vi "Configuration--FGV.vi"(7 "Functional Global Action":T4, 9 "Module Number":i32, 10 "Module Configuration In":T2, 11 "Carrier Configuration In":T1) -> (2 "Module Configuration Out":T2, 3 "Carrier Configuration Out":T1)   [LabVIEW 2017, in "Communications Library.lvlib"]
doc: "Functional gloabl variable, which stores the current configuration of the DTACQ device. \n\nNote: Writting the carrier configuration will also replace the module configurations."
uses:
  Communications Library.lvlib
  Typedefs/Functional Global Variable Action--Enum.ctl
  Typedefs/DTACQ Module Carrier Configuration--Cluster.ctl
  Typedefs/DTACQ Module Configuration--Cluster.ctl
  Typedefs/DTACQ Device Type--Enum.ctl
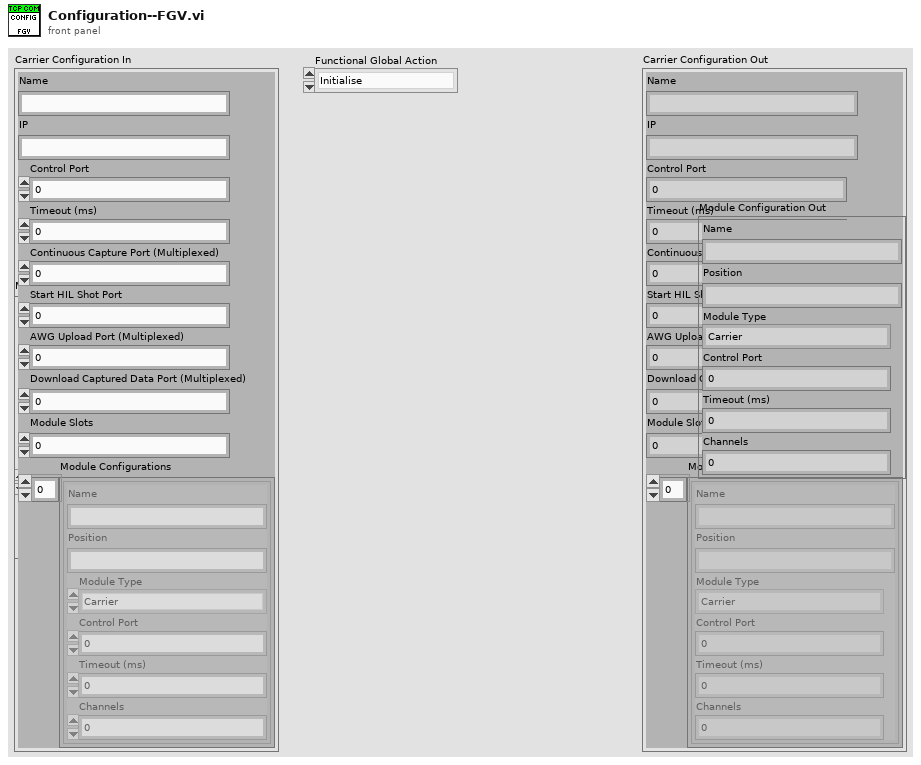
[diagram p1: front panel]
types:
  T1 = typedef "Communications Library.lvlib/DTACQ Module Carrier Configuration--Cluster.ctl" = cluster{"Name":string, "IP":string, "Control Port":i32, "Timeout (ms)":i32, "Continuous Capture Port (Multiplexed)":i32, "Start HIL Shot Port":i32, "AWG Upload Port (Multiplexed)":i32, "Download Captured Data Port (Multiplexed)":i32, "Module Slots":i32, "Module Configurations":T2[]}
  T2 = typedef "Communications Library.lvlib/DTACQ Module Configuration--Cluster.ctl" = cluster{"Name":string, "Position":string, "Module Type":T3, "Control Port":i32, "Timeout (ms)":i32, "Channels":i32}
  T3 = typedef "Communications Library.lvlib/DTACQ Device Type--Enum.ctl" = enum16{"Carrier", "Analog In Module", "Analog Out Module", "Generic Module"}
  T4 = typedef "Communications Library.lvlib/Functional Global Variable Action--Enum.ctl" = enum16{"Initialise", "Write Module Config", "Write Carrier Config", "Read"}
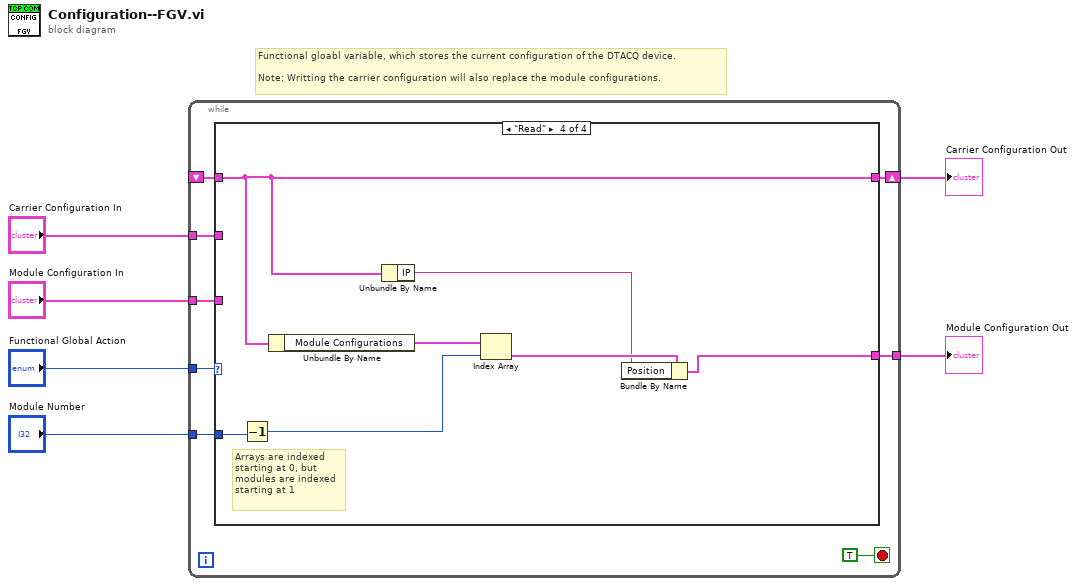
[diagram p0: block diagram]
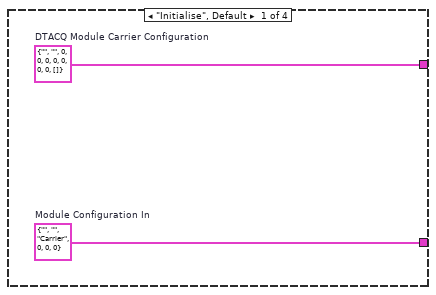
[diagram p2: hidden frame]
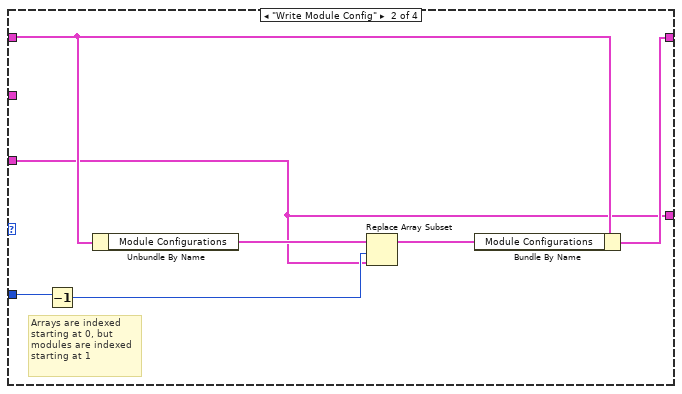
[diagram p3: hidden frame]
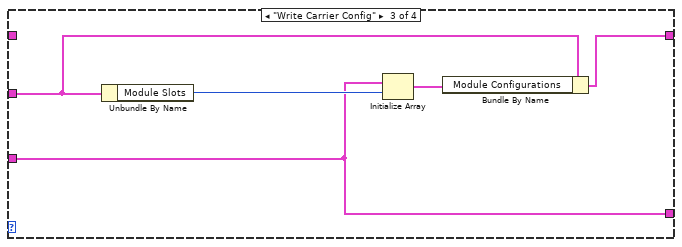
[diagram p4: hidden frame]
diagram:
  # "Functional gloabl variable, which stores the current configuration of the DTACQ device.  \n\nNote: Writting the carrier configuration will also replace the module configurations."
  n1 = while {
    tunnel: "Functional Global Action" -> [w14]
    shift-right: [w13] -> w4
    shift-left: _ -> [w12]
    tunnel: "Module Number" -> [w11]
    tunnel: [w10] -> w3
    tunnel: "Module Configuration In" -> [w9]
    tunnel: "Carrier Configuration In" -> [w8]
    stop <- TRUE stop-if-true
    n2 = case shown="\"Read\"" w14 {
      tunnel: [w16 w22 w25 w32] -> w13
      tunnel: w12 -> [_ w23 _ w32]
      tunnel: w11 -> [_ w20 _ w34]
      tunnel: [w15 w18 w24 w29] -> w10
      tunnel: w9 -> [_ w18 w24 _]
      tunnel: w8 -> [_ _ w26 _]
      frame "Initialise", Default {
        w15 = T2 {"Name"="", "Position"="", "Module Type"=enum."Carrier", "Control Port"=0, "Timeout (ms)"=0, "Channels"=0}  # Module Configuration In
        w16 = T1 {"Name"="", "IP"="", "Control Port"=0, "Timeout (ms)"=0, "Continuous Capture Port (Multiplexed)"=0, "Start HIL Shot Port"=0, "AWG Upload Port (Multiplexed)"=0, "Download Captured Data Port (Multiplexed)"=0, "Module Slots"=0, "Module Configurations"=[]}  # DTACQ Module Carrier Configuration
      }
      frame "Write Module Config" {
        # "Arrays are indexed \nstarting at 0, but \nmodules are indexed\nstarting at 1"
        n3 = Decrement(x=w20) -> (x-1=w19:i32)
        n4 = Unbundle By Name(w23) -> ("Module Configurations"=w21:T2[])
        n5 = Replace Array Subset(array=w21, new element=w18, index=w19) -> (w17:T2[])
        n6 = Bundle By Name(cluster=w23, "Module Configurations"=w17) -> (w22:T1)
      }
      frame "Write Carrier Config" {
        n7 = Unbundle By Name(w26) -> ("Module Slots"=w28:i32)
        n8 = Initialize Array(w24, w28) -> (w27:T2[])
        n9 = Bundle By Name(cluster=w26, "Module Configurations"=w27) -> (w25:T1)
      }
      frame "Read" {
        # "Arrays are indexed \nstarting at 0, but \nmodules are indexed\nstarting at 1"
        n10 = Decrement(x=w34) -> (x-1=w33:i32)
        n11 = Unbundle By Name(w32) -> ("Module Configurations"=w35:T2[])
        n12 = Unbundle By Name(w32) -> ("IP"=w30:string)
        n13 = Index Array(array=w35, index=w33) -> (element=w31:T2)
        n14 = Bundle By Name(cluster=w31, "Position"=w30) -> (w29:T2)
      }
    }
  }
  "Carrier Configuration Out" <- w4
  "Module Configuration Out" <- w3
